vi "PicoScope3000aPowerSource.vi"(6 "USB 3.0 on non-USB 3.0 port control":bool=TRUE, 7 "Mode":u16(ring) items=["Dialog On Error", "no dialog - CloseUnit and Stop", "no dialog - Continue", "no dialog - Stop"], 8 "USB Powered control":bool=TRUE, 9 "handle in":i16, 10 "PICO STATUS IN":u32 format="%#.0f", 11 "error in (no error)":errorcluster) -> (0 "USB Powered":bool=TRUE, 1 "handle out":i16, 2 "PICO STATUS OUT":u32, 3 "error out":errorcluster, 4 "USB 3.0 on non-USB 3.0 Port":bool=TRUE)   [LabVIEW 2010]
uses:
  ps3000a.dll
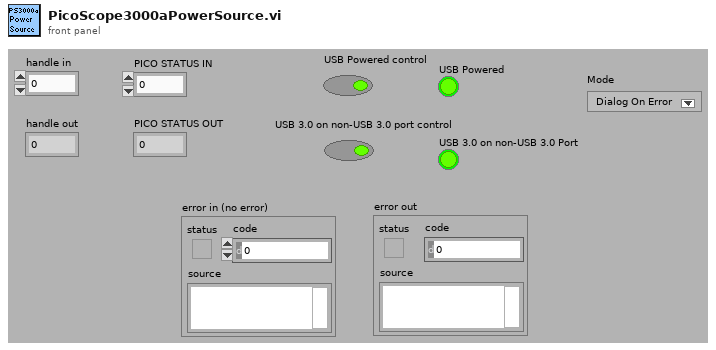
[diagram p1: front panel]
types:
  T1 = cluster{"status":bool, "code":u32, "source":string}
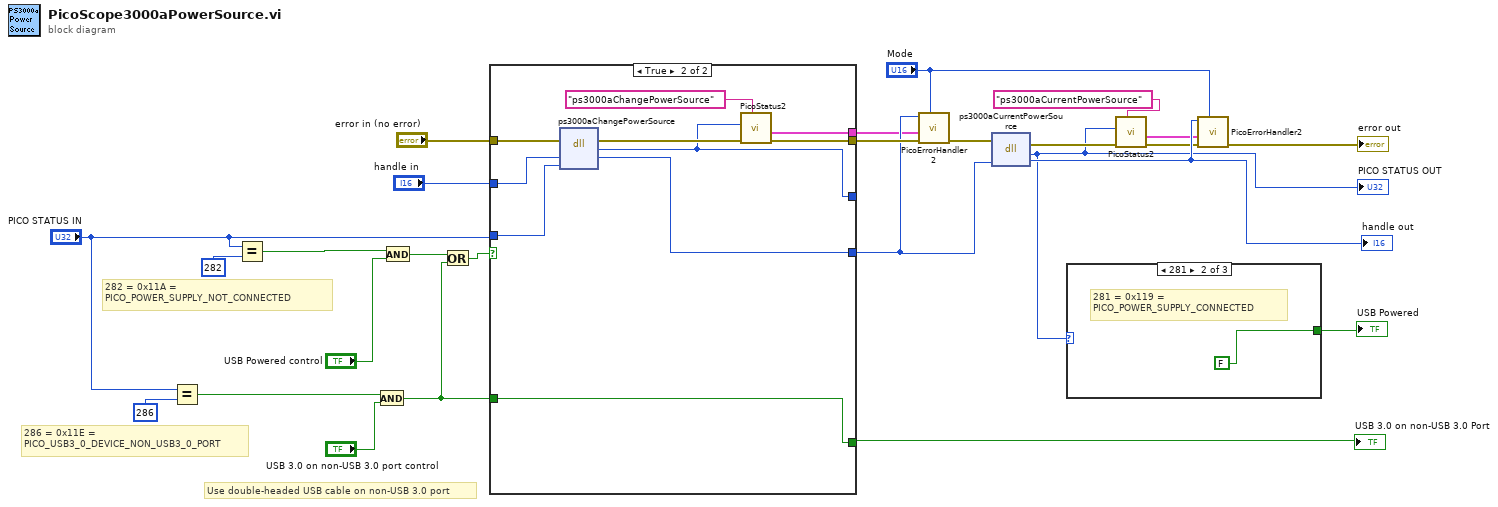
[diagram p0: block diagram]
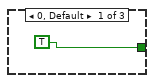
[diagram p2: hidden frame]
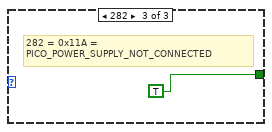
[diagram p3: hidden frame]
diagram:
  # "Use double-headed USB cable on non-USB 3.0 port"
  # "286 = 0x11E = \nPICO_USB3_0_DEVICE_NON_USB3_0_PORT"
  # "282 = 0x11A = \nPICO_POWER_SUPPLY_NOT_CONNECTED"
  n1 = Equal?(x="PICO STATUS IN", y=u32 286) -> (x = y?=w18:bool)
  n2 = Equal?(x="PICO STATUS IN", y=u32 282) -> (x = y?=w25:bool)
  n3 = And(x=w18, y="USB 3.0 on non-USB 3.0 port control") -> (x .and. y?=w8:bool)
  n4 = And(x=w25, y="USB Powered control") -> (x .and. y?=w15:bool)
  n5 = Or(x=w15, y=w8) -> (x .or. y?=w16:bool)
  n6 = case shown="True" w16 {
    tunnel: "PICO STATUS IN" -> [w30 w39]
    tunnel: [w30 w33] -> _
    tunnel: [w29 w32] -> w13
    tunnel: "error in (no error)" -> [w29 w40]
    tunnel: "handle in" -> [w28 w38]
    tunnel: [w27 w36] -> w19
    tunnel: [w28 w37] -> w11
    tunnel: w8 -> [w27 w36]
    tunnel: [_ w31] -> w1
    frame False {
    }
    frame True {
      n7 = dll-call lib="ps3000a.dll" fn="ps3000aChangePowerSource"(error in=w40, "handle"=w38, "powerSource"=w39) -> (error out=w35:errorcluster, "PICO_STATUS"=w33:u32, "handle"=w37:i16)  [unwired: 3 in, 1 out]
      n8 = call "PicoStatus2.vi"("PICO source"="ps3000aChangePowerSource" ("source"), "Error in"=w35, "PICO STATUS"=w33) -> ("error out"=w32:errorcluster, "PICO_STATUS out"=w31:T1)  [unwired: 5 in]
    }
  }
  "USB 3.0 on non-USB 3.0 Port" <- w19
  n9 = call "PicoErrorHandler2.vi"("Mode"="Mode", "error in (no error)"=w13, "PICO_STATUS in"=w1, "handle In"=w11) -> ("error out"=w12:errorcluster)  [unwired: 7 in]
  n10 = dll-call lib="ps3000a.dll" fn="ps3000aCurrentPowerSource"(error in=w12, "handle"=w11) -> (error out=w4:errorcluster, "PICO_STATUS"=w3:u32, "handle"=w10:i16)  [unwired: 2 in, 1 out]
  "PICO STATUS OUT" <- w3
  "handle out" <- w10
  n11 = case shown="281" w3 {
    tunnel: [TRUE FALSE TRUE] -> w14
    frame 0, Default {
    }
    frame 281 {
      # "281 = 0x119 = \nPICO_POWER_SUPPLY_CONNECTED"
    }
    frame 282 {
      # "282 = 0x11A = \nPICO_POWER_SUPPLY_NOT_CONNECTED"
    }
  }
  "USB Powered" <- w14
  n12 = call "PicoStatus2.vi"("PICO source"="ps3000aCurrentPowerSource" ("source"), "Error in"=w4, "PICO STATUS"=w3) -> ("error out"=w6:errorcluster, "PICO_STATUS out"=w5:T1)  [unwired: 5 in]
  n13 = call "PicoErrorHandler2.vi"("Mode"="Mode", "error in (no error)"=w6, "PICO_STATUS in"=w5, "handle In"=w10) -> ("error out"=→"error out":errorcluster)  [unwired: 7 in]
